vi "FA_ConvertFromINIConfig.vi"(8 "Error In":errorcluster, 11 "XML String":string) -> (0 "Error Out":errorcluster, 3 "Config":T1)   [LabVIEW 2013, in "FA_INI.lvlib"]
doc: "Converts an XML string describing an INI configuration into a LabVIEW typedef"
uses:
  FA_INI.lvlib
  FA_INIconfig.ctl
  FA_INI.ctl
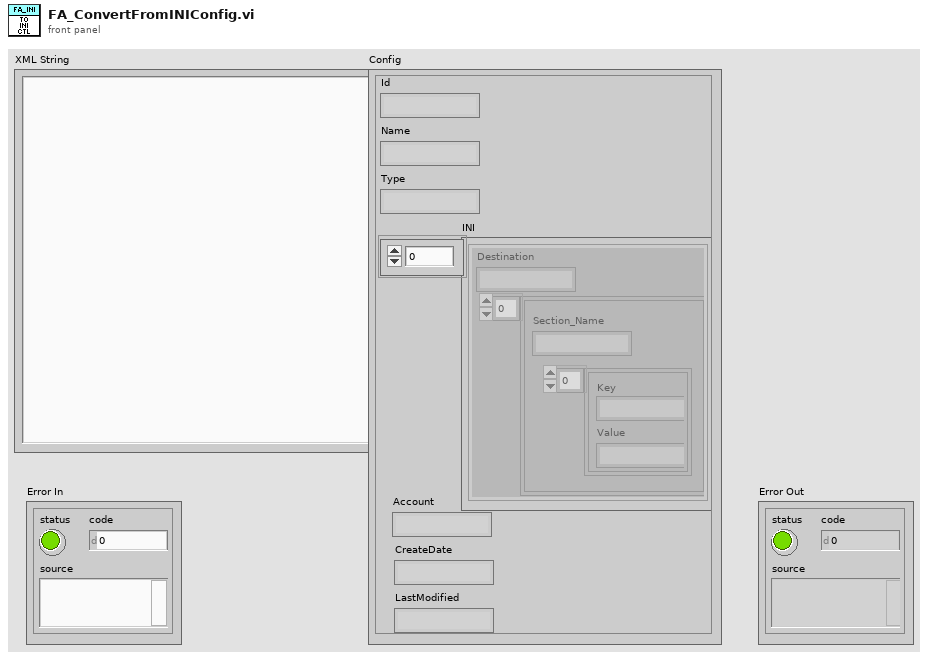
[diagram p1: front panel]
types:
  T1 = typedef "FA_INI.lvlib/FA_INIconfig.ctl" = cluster{"Id":string, "Name":string, "Type":string, "INI":T2, "Account":string, "CreateDate":string, "LastModified":string}
  T2 = typedef "FA_INI.ctl" = cluster{"Destination":string, "Section":cluster{"Section_Name":string, "Token":cluster{"Key":string, "Value":string}[]}[]}[]
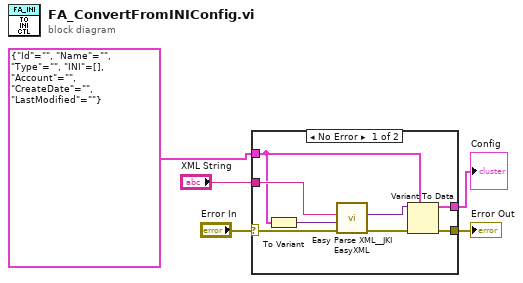
[diagram p0: block diagram]
diagram:
  n1 = case shown="No Error" "Error In" {
    selector: "Error In" -> [w8 w15]
    tunnel: "XML String" -> [w13 _]
    tunnel: [w9 w15] -> w3
    tunnel: T1 {"Id"="", "Name"="", "Type"="", "INI"=[], "Account"="", "CreateDate"="", "LastModified"=""} ("Config") -> [w7 w14]
    tunnel: [w6 w14] -> w2
    frame No Error {
      n2 = To Variant(anything=w7) -> (Variant=w12:variant)
      n3 = call <vilib>:"Easy Parse XML__JKI EasyXML.vi"("error in (no error)"=w8, "LabVIEW Data (Type)"=w12, "XML String"=w13) -> ("error out"=w11:errorcluster, "LabVIEW Data"=w10:variant)  [unwired: 7 in]
      n4 = Variant To Data(error in=w11, type=w7, Variant=w10) -> (data=w6:T1, error out=w9:errorcluster)
    }
    frame Error {
    }
  }
  "Error Out" <- w3
  "Config" <- w2
